vi "Untitled 2.vi"() -> ()   [LabVIEW 2020]
uses:
  Disp_Parameter.ctl
panel:
  out "Parameter":T1
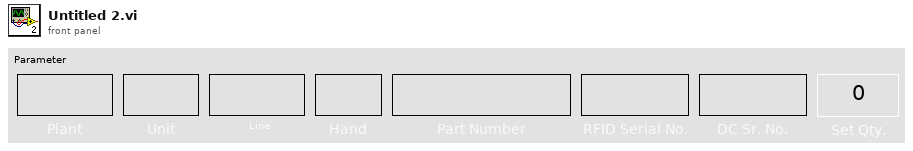
[diagram p1: front panel]
types:
  T1 = typedef "Disp_Parameter.ctl" = cluster{"Plant":string, "Unit":string, "Line":string, "Hand":string, "Part Number":string, "RFID Serial No.":string, "DC Sr. No.":string, "Set Qty.":i32}
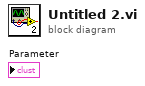
[diagram p0: block diagram]
diagram:
